vi "Draw Text in Rect.vi"(4 "BG color(transparent)":u32(colorbox)=16777216, 5 "[user-specified font]":T3={"Font Name:"="", "Size"=12, "Strikeout?"=FALSE, "Italic?"=FALSE, "Underline?"=FALSE, "Outline?"=FALSE, "Shadow?"=FALSE, "Bold?"=FALSE}, 6 "text color(black)":u32(colorbox), 7 "desired font(Application)":T2(ring)=enum."Application Font", 8 "text":string, 9 "rect":T4, 10 "text orientation":T1(ring), 11 "picture":picture) -> (3 "new picture":picture)   [LabVIEW 2021, in "Picture Pixel Fonts.lvlib"]
doc: "<p>Draws a string into a picture.</p>"
uses:
  <vilib>/LabVIEW Icon API/Pixel Fonts/Picture Pixel Fonts.lvlib
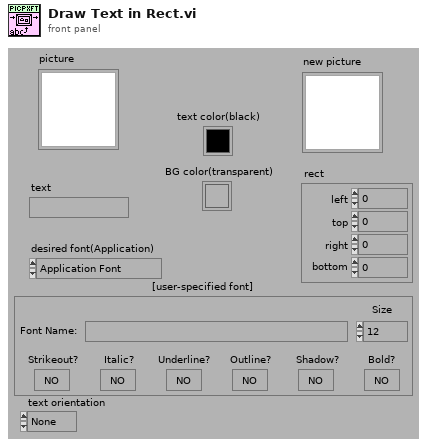
[diagram p1: front panel]
types:
  T1 = enum16{"None", "Stacked", "Clockwise", "Counterclockwise"}
  T2 = enum16{"User-specified Font", "Application Font", "System Font", "Dialog Font"}
  T3 = cluster{"Font Name:":string, "Size":i16, "Strikeout?":bool, "Italic?":bool, "Underline?":bool, "Outline?":bool, "Shadow?":bool, "Bold?":bool}
  T4 = cluster{"left":i16, "top":i16, "right":i16, "bottom":i16}
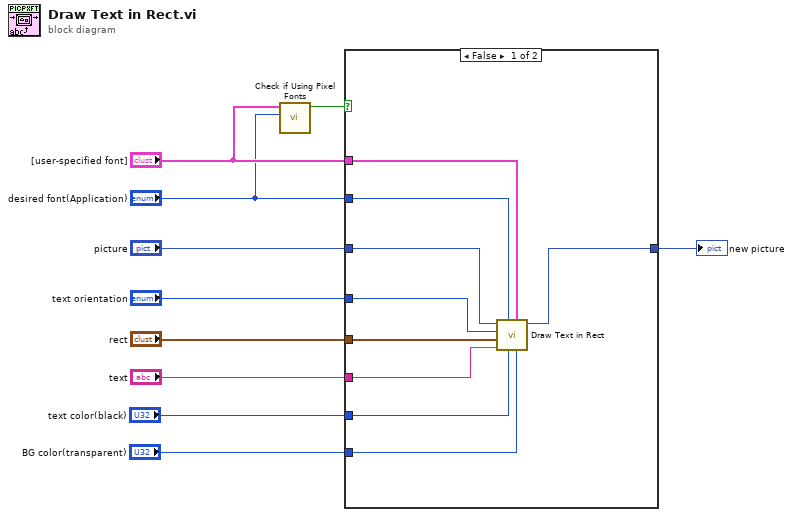
[diagram p0: block diagram]
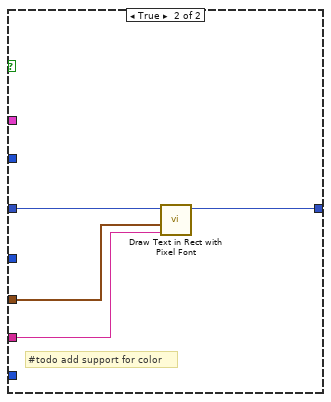
[diagram p2: hidden frame]
diagram:
  n1 = call <vilib>:"Check if Using Pixel Fonts.vi"("desired font(Application)"="desired font(Application)", "[user-specified font]"="[user-specified font]") -> ("use_pixel_fonts"=w1:bool)  [unwired: 9 in]
  n2 = case shown="False" w1 {
    tunnel: "text" -> [w19 w20]
    tunnel: "rect" -> [w18 w21]
    tunnel: "text orientation" -> [w17 _]
    tunnel: "picture" -> [w16 w23]
    tunnel: [w15 w22] -> w6
    tunnel: "BG color(transparent)" -> [w14 _]
    tunnel: "text color(black)" -> [w13 _]
    tunnel: "[user-specified font]" -> [w12 _]
    tunnel: "desired font(Application)" -> [w11 _]
    frame False {
      n3 = call <vilib>:"Draw Text in Rect.vi"("BG color(transparent)"=w14, "[user-specified font]"=w12, "text color(black)"=w13, "desired font(Application)"=w11, "text"=w19, "rect"=w18, "text orientation"=w17, "picture"=w16) -> ("new picture"=w15:picture)  [unwired: 3 in]
    }
    frame True {
      # "#todo add support for color"
      n4 = call <vilib>:"Draw Text in Rect with Pixel Font.vi"("string"=w20, "Rectangle"=w21, "picture"=w23) -> ("new picture"=w22:picture)  [unwired: 8 in]
    }
  }
  "new picture" <- w6
